vi "Register Process.vi"(6 "Forces Self to Run (F)":bool, 7 "Parent Call":T1, 8 "error in (no error)":errorcluster, 9 "Process Name (optional)":string, 11 "SMO":refnum<class "SMO.lvclass">) -> (0 "error out":errorcluster, 3 "SMO out":refnum<class "SMO.lvclass">)   [LabVIEW 2019, in "SMO.lvclass"]
doc: "Philosophy of Registration of SMOs\n=========================\nOverriding \"Process.vi\" is mandatory (Must Call Parent) to allow the framework to achieve necessary housekeeping functionality.\nThere are two ways the developer can override a process: a) by extending its functionalities (EXTENSION) or b) by overwriting its functionalities (OVERWRITE).\nEven if the parent method has to be called, the framework allows the developer to request that its parent process not run (overwriting).\n\nAt this point, it becomes the responsibility of the parent process to decide if it should comply with this request or ignore it. If it chooses to ignore its child's request,\nthe process will be extended. This is meant to allow a process to do critical functions necessary to its performance even if the child requests to overwrite it.\n\nIn a nutshell, each process can decide at runtime if it allows itself to be overwritten or simply extended by a more specific implementation.JKI State Machine Objects (SMO) 1.3.0.56\nJKI - JKI\nCopyright (c) 2017, JKI"
uses:
  SMO.lvclass
  Typedefs/Parent Call--Enum.ctl
  SMO.lvclass/SMO.ctl
panel:
  # "For instructions on how to use the JKI State Machine Objects, examples and video tutorials, visit:\nhttp://jki.net/state-machine-objects/\n\nJKI State Machine Objects™\nhttp://jki.net/state-machine-objects/\nCopyright (C) 2005-2015, JKI <info@jki.net>\nALL RIGHTS RESERVED"
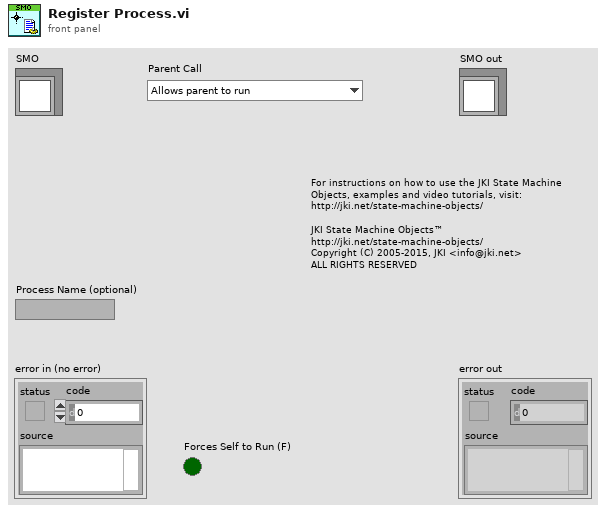
[diagram p1: front panel]
types:
  T1 = typedef "SMO.lvclass/Parent Call--Enum.ctl" = enum16{"Allows parent to run", "Does not request parent to run"}
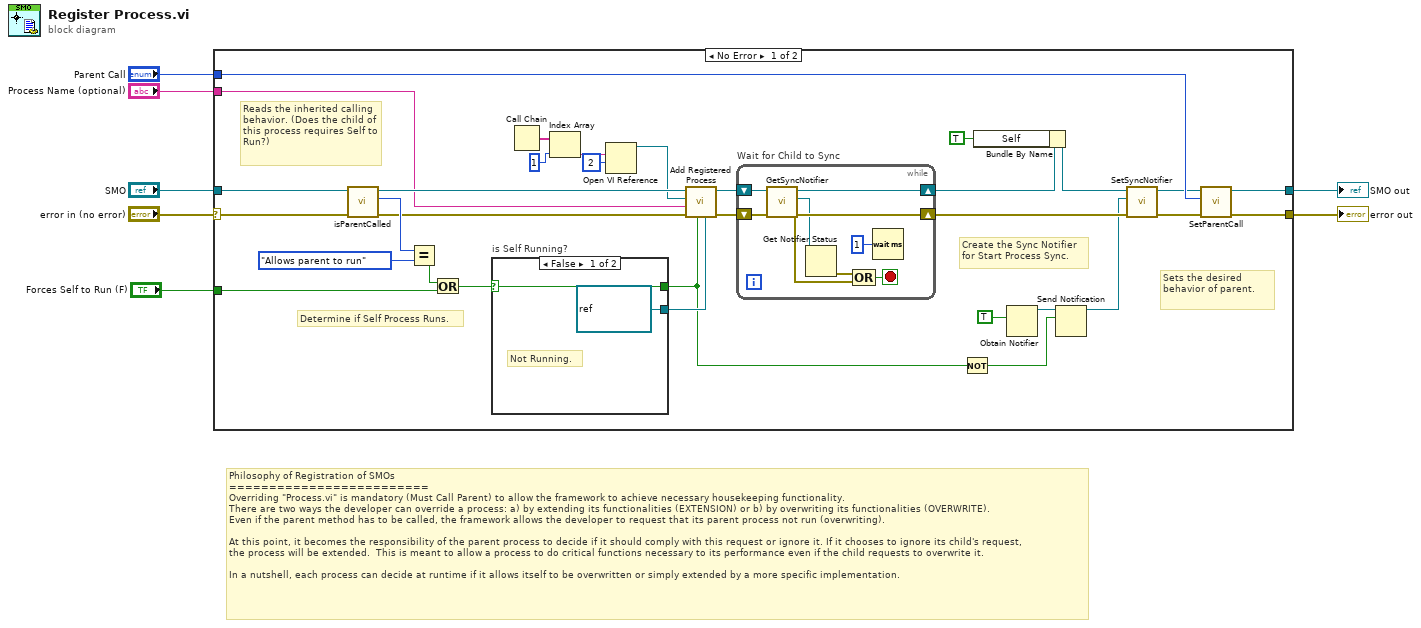
[diagram p0: block diagram]
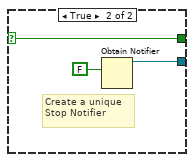
[diagram p2: hidden frame]
diagram:
  # "Philosophy of Registration of SMOs\n=========================\nOverriding \"Process.vi\" is mandatory (Must Call Parent) to allow the framework to achieve necessary housekeeping functionality.\nThere are two ways the developer can override a process: a) by extending its functionalities (EXTENSION) or b) by overwriting its functionalities (OVERWRITE).\nEven if the parent method has to be called, the framework allows the developer to request that its parent process not run (overwriting).\n\nAt this point, it becomes the responsibility of the parent process to decide if it should comply with this request or ignore it. If it chooses to ignore its child's request,\nthe process will be extended.  This is meant to allow a process to do critical functions necessary to its performance even if the child requests to overwrite it.\n\nIn a nutshell, each process can decide at runtime if it allows itself to be overwritten or simply extended by a more specific implementation."
  n1 = case shown="No Error" "error in (no error)" {
    selector: "error in (no error)" -> [w21 w53]
    tunnel: "SMO" -> [w22 w54]
    tunnel: [w32 w54] -> w6
    tunnel: [w31 w53] -> w4
    tunnel: "Process Name (optional)" -> [w23 _]
    tunnel: "Parent Call" -> [w38 _]
    tunnel: "Forces Self to Run (F)" -> [w36 _]
    frame No Error {
      # "Create the Sync Notifier\nfor Start Process Sync."
      # "Determine if Self Process Runs."
      # "Sets the desired behavior of parent."
      # "Reads the inherited calling behavior. (Does the child of this process requires Self to Run?)"
      n2 = call "isParentCalled.vi"("error in (no error)"=w21, "SMO in"=w22) -> ("error out"=w25:errorcluster, "Parent Call"=w39:T1, "SMO out"=w26:refnum<class "SMO.lvclass">)  [unwired: 7 in]
      n3 = Equal?(x=w39, y=Parent_Call--Enum."Allows parent to run") -> (x = y?=w37:bool)
      n4 = Or(x=w37, y=w36) -> (x .or. y?=w19:bool)
      n5 = case "is Self Running?" shown="False" w19 {
        selector: w19 -> [w49 w51]
        tunnel: [refnum<notifier> refnum ("notifier out") w52] -> w20
        tunnel: [w49 w51] -> w10
        frame False {
          # "Not Running."
        }
        frame True {
          # "Create a unique Stop Notifier"
          n6 = Obtain Notifier(notification data type=FALSE) -> (notifier out=w52:refnum<notifier>)  [unwired: 3 in, 2 out]
        }
      }
      n7 = Call Chain() -> (call chain=w27:string[])
      n8 = Index Array(array=w27, index=1 ("Index")) -> (element=w29:string)
      n9 = Open VI Reference(vi path=w29, options=2) -> (vi reference=w24:refnum<vi>)  [unwired: 4 in, 1 out]
      n10 = call "Add Registered Process.vi"("Sync Notifier"=w20, "Process Runs (T)"=w10, "error in (no error)"=w25, "Process Name (Optional)"=w23, "Process VI (Static VI Ref)"=w24, "SMO"=w26) -> ("error out"=w17:errorcluster, "SMO out"=w18:refnum<class "SMO.lvclass">)  [unwired: 4 in]
      n11 = while "Wait for Child to Sync" {
        shift-right: [w46] -> w14
        shift-left: w18 -> [w47]
        shift-right: [w43] -> w16
        shift-left: w17 -> [w45]
        stop <- w44 stop-if-true
        n12 = call "GetSyncNotifier.vi"("error in (no error)"=w45, "SMO in"=w47) -> ("error out"=w43:errorcluster, "Sync Notifier"=w41:refnum<notifier>, "SMO out"=w46:refnum<class "SMO.lvclass">)  [unwired: 7 in]
        n13 = Get Notifier Status(notifier=w41) -> (error out=w40:errorcluster)  [unwired: 1 in, 4 out]
        n14 = Compound Arithmetic op=OR(w40, w43) -> (w44:bool)
        n15 = Wait (ms)(milliseconds to wait=u32 1) -> ()  [unwired: 1 out]
      }
      n16 = Not(x=w10) -> (.not. x?=w9:bool)
      n17 = Bundle By Name(cluster=w14, "Self"=TRUE ("Reserved.Self")) -> (w13:refnum<class "SMO.lvclass">)
      n18 = Obtain Notifier(notification data type=TRUE) -> (notifier out=w11:refnum<notifier>)  [unwired: 3 in, 2 out]
      n19 = Send Notification(notification=w9, notifier=w11) -> (notifier out=w8:refnum<notifier>)  [unwired: 1 in, 1 out]
      n20 = call "SetSyncNotifier.vi"("error in (no error)"=w16, "Sync Notifier"=w8, "SMO in"=w13) -> ("error out"=w33:errorcluster, "SMO out"=w34:refnum<class "SMO.lvclass">)  [unwired: 7 in]
      n21 = call "SetParentCall.vi"("error in (no error)"=w33, "Parent Call"=w38, "SMO in"=w34) -> ("error out"=w31:errorcluster, "SMO out"=w32:refnum<class "SMO.lvclass">)  [unwired: 7 in]
    }
    frame Error {
    }
  }
  "error out" <- w4
  "SMO out" <- w6
